vi "Process.vi"(8 "error in":errorcluster, 11 "Sequence Experiment UI":refnum<class "Sequence Experiment UI.lvclass">) -> (0 "error out":errorcluster, 3 "Sequence Experiment UI out":refnum<class "Sequence Experiment UI.lvclass">)   [LabVIEW 2019, in "Sequence Experiment UI.lvclass"]
doc: "---------------------------------------------------------------\nJKI State Machine Objects™\nhttp://jki.net/state-machine-objects/\nCopyright (C) 2005-2015, JKI <info@jki.net>\nALL RIGHTS RESERVEDJKI State Machine Objects (SMO) 1.0.0.5\nJKI - JKI\nCopyright (c) 2016, JKI"
uses:
  Sequence Experiment UI.lvclass
  <vilib>/JKI/JKI SMO/SMO/SMO.lvclass
  <vilib>/JKI/JKI SMO/SMO.UI/SMO.UI.lvclass
  <userlib>/LevyLab/Instrument Framework/SMOs/Instrument/Instrument.lvclass
  C:/Program Files (x86)/National Instruments/LabVIEW 2019/user.lib/LevyLab/Instrument Framework/SMOs/Instrument UI/Instrument UI.lvclass
  C:/Program Files (x86)/National Instruments/LabVIEW 2019/vi.lib/JKI/JKI SMO/SMO.UI/SMO.UI.lvclass
  C:/Program Files (x86)/National Instruments/LabVIEW 2019/vi.lib/JKI/JKI SMO/SMO/SMO.lvclass
  <userlib>/LevyLab/Instrument Framework/SMOs/Instrument UI/Instrument UI.lvclass
  8548cf1d-4249-4658-ae96-b7b094251154.vi
panel:
  out "Numeric":u32
  out "Instrument Response":dbl
  in  "Set Parameter":bool
  in  "Parameter":dbl
  in  "STOP":bool
  out "SMO string":string
  out "SMO Boolean":bool
  out "Logger SMO":dbl
  out "Levy 1":dbl
  # "#todo\nmake UI here. maybe include a nice picture of the hardware?"
  # "#todo\nadd buttons to do stuff (e.g., change a setting)\nButtons should trigger an event"
  # "#todo\nresize this box if you want your UI to be different size"
  # "SMO UI Template"
  # "For instructions on how to use the JKI State Machine Objects, examples and video tutorials, visit:\nhttp://jki.net/state-machine-objects/\n\nJKI State Machine Objects™\nhttp://jki.net/state-machine-objects/\nCopyright (C) 2005-2015, JKI <info@jki.net>\nALL RIGHTS RESERVED"
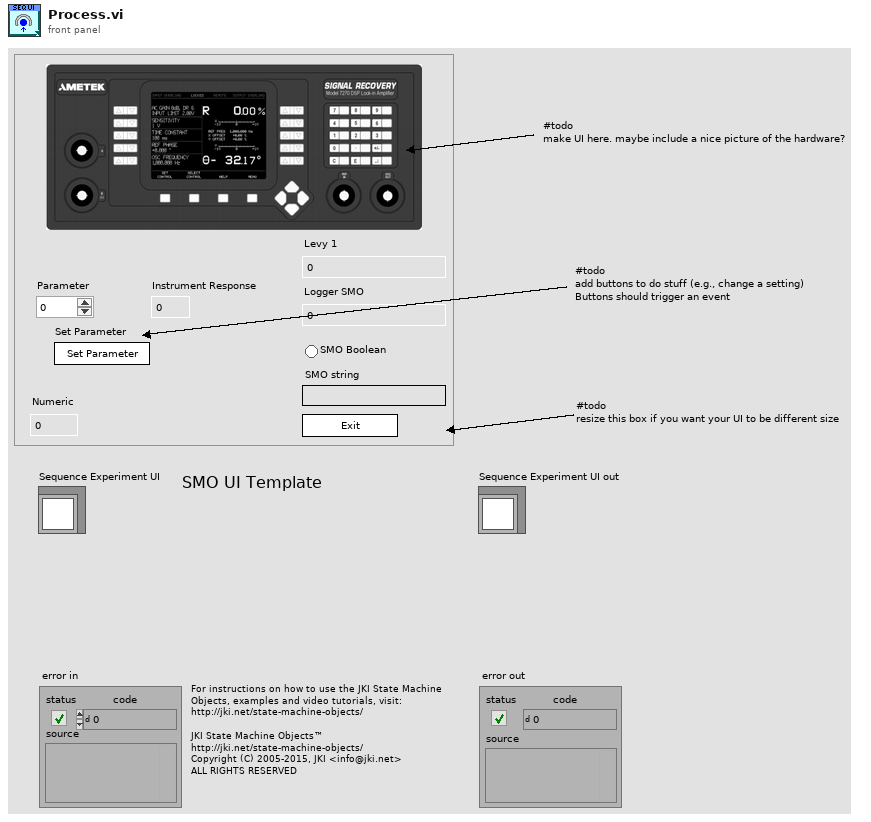
[diagram p1: front panel]
types:
  T1 = enum32{"invalid app kind", "Development System", "Run Time System", "Student Edition", "Embedded LabVIEW", "Evaluation", "Custom"}
  T2 = enum32{"Invalid", "Standard", "Closed", "Hidden", "Minimized", "Maximized"}
  T3 = cluster{"Core":cluster{"Current VI Reference":refnum<vi>, "Close Panel on Exit?":bool, "error":errorcluster}, "Instrument UI":refnum<class "Sequence Experiment UI.lvclass">, "Instrument":refnum<class "Instrument.lvclass">, "getAll":cluster{"Levy 1":dbl, "Logger SMO":dbl, "SMO Boolean":bool, "SMO String":string}, "Parameter":dbl}
  T4 = cluster{"Levy 1":dbl, "Logger SMO":dbl, "SMO Boolean":bool, "SMO String":string}
  T5 = cluster{"Current VI Reference":refnum<vi>, "Close Panel on Exit?":bool, "error":errorcluster}
  T6 = typedef "SMO.lvclass/Protected Events.ctl" = cluster{"StopProcesses":refnum<user-event>, "AbortProcesses":refnum<user-event>, "Config Changed":refnum<user-event>, "Dependency":refnum<user-event>}
  T7 = typedef "Instrument.lvclass/PublicEvents--Cluster.ctl" = cluster{"MessageFromProcess":refnum<user-event>}
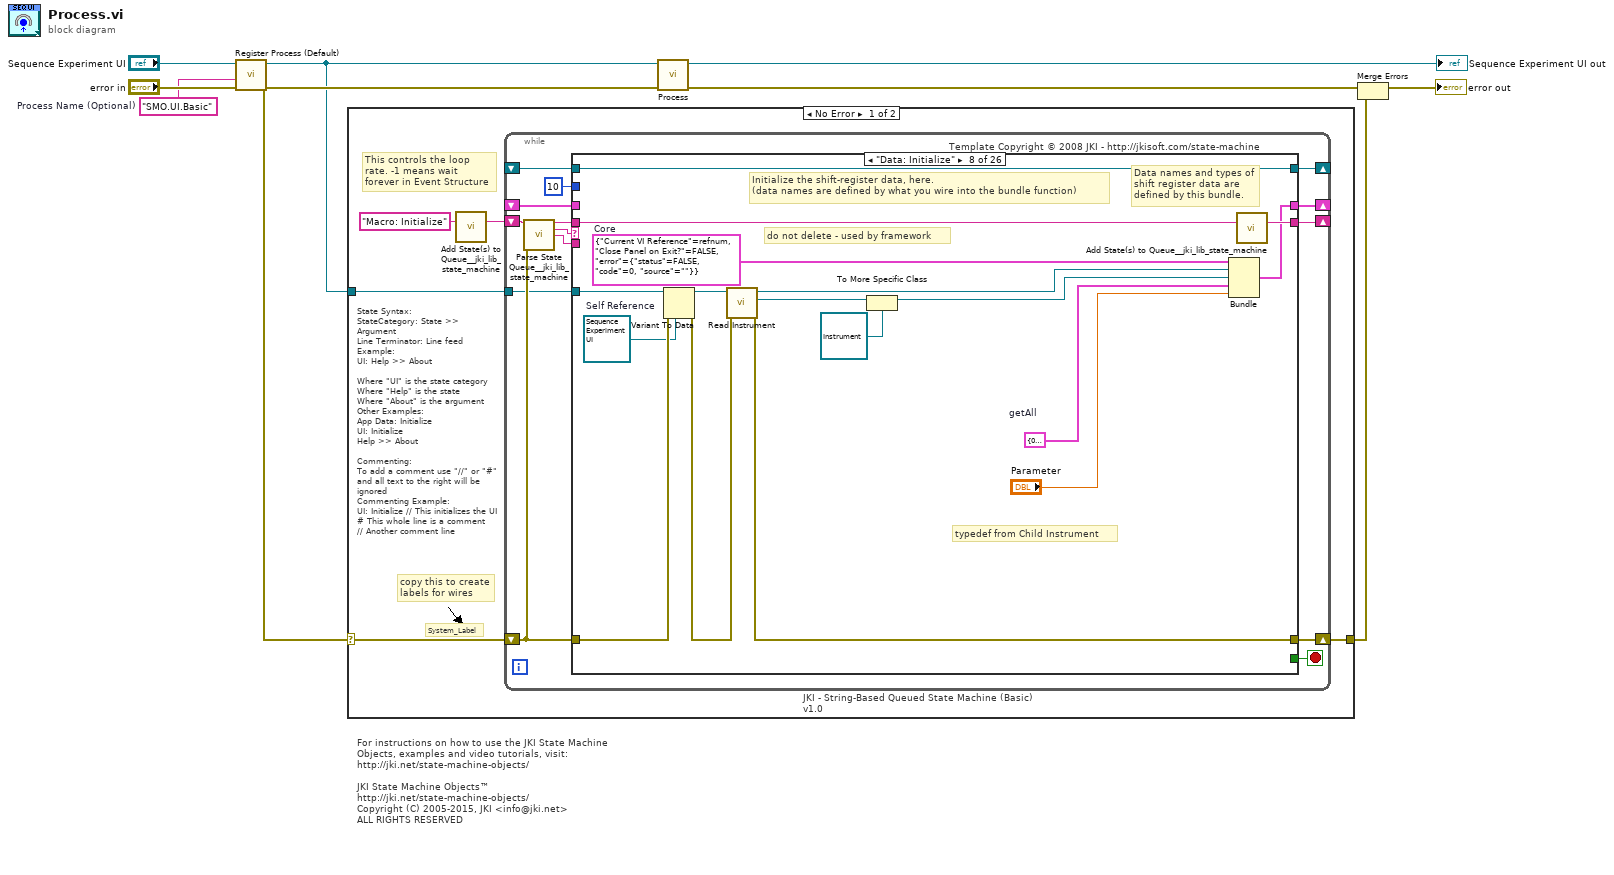
[diagram p0: block diagram]
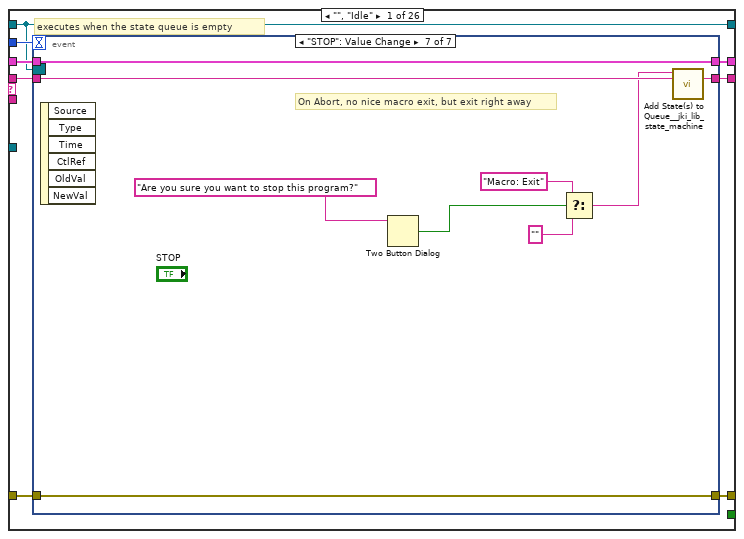
[diagram p2: hidden frame]
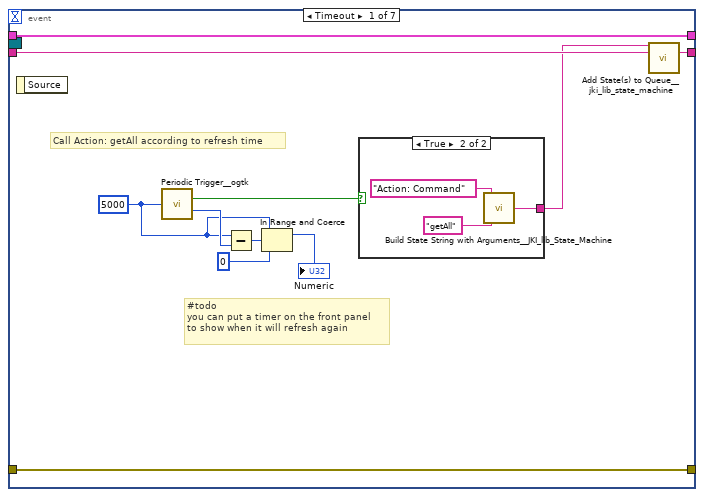
[diagram p3: hidden frame]
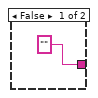
[diagram p4: hidden frame]
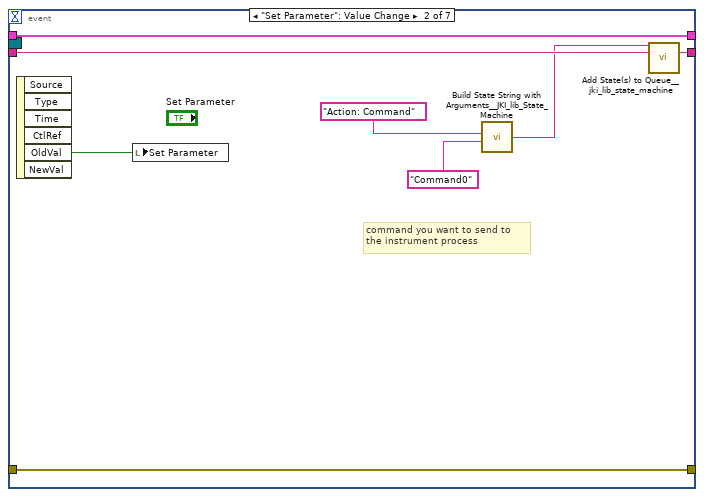
[diagram p5: hidden frame]
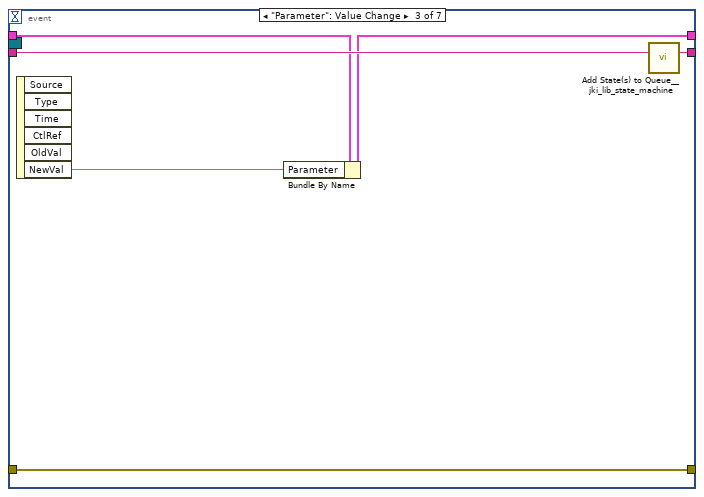
[diagram p6: hidden frame]
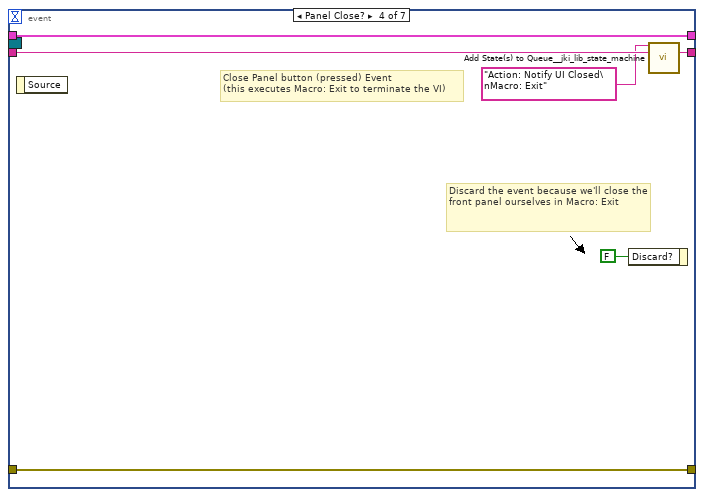
[diagram p7: hidden frame]
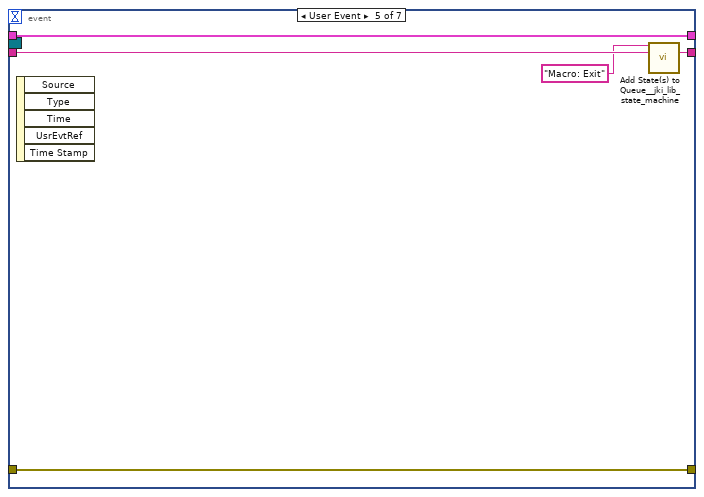
[diagram p8: hidden frame]
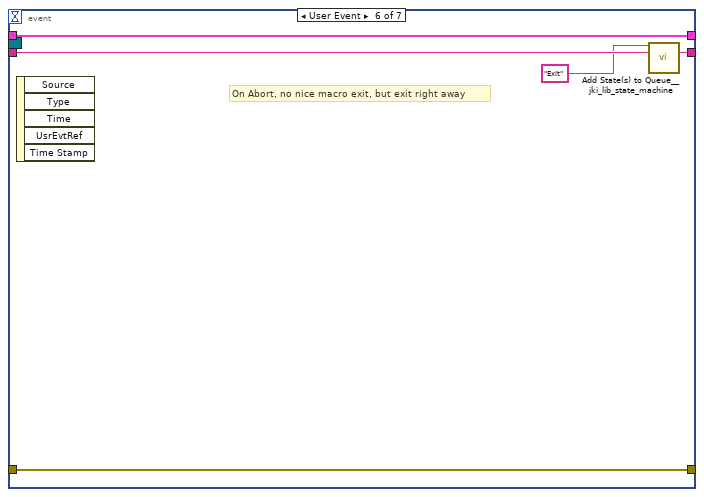
[diagram p9: hidden frame]
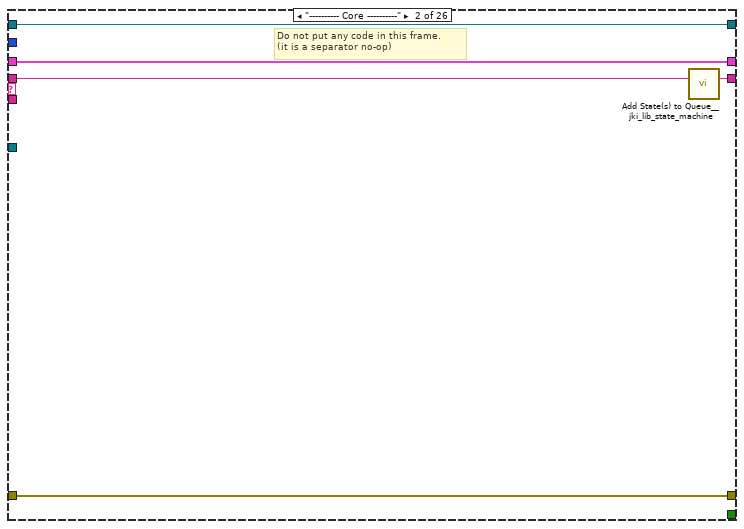
[diagram p10: hidden frame]
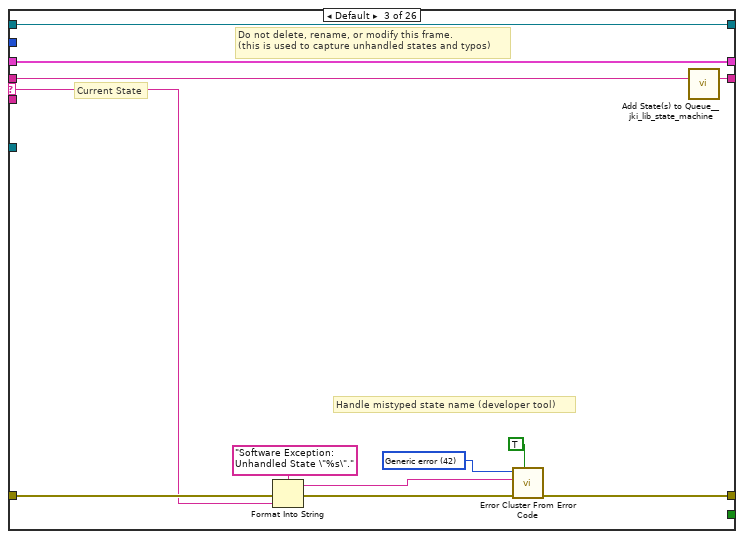
[diagram p11: hidden frame]
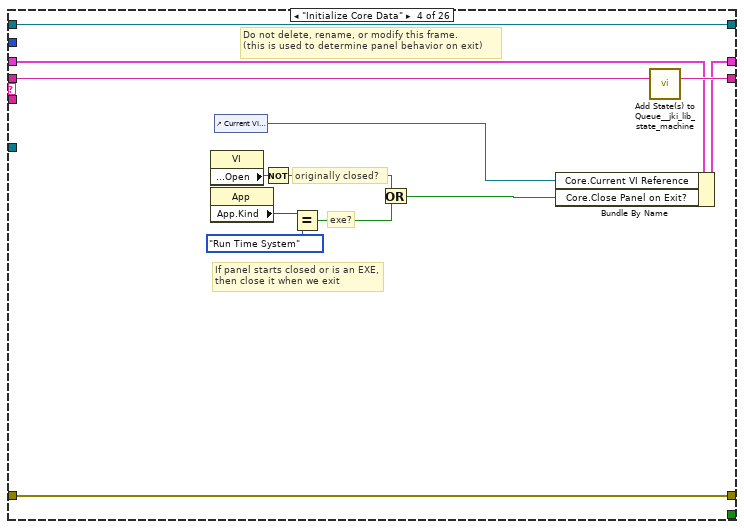
[diagram p12: hidden frame]
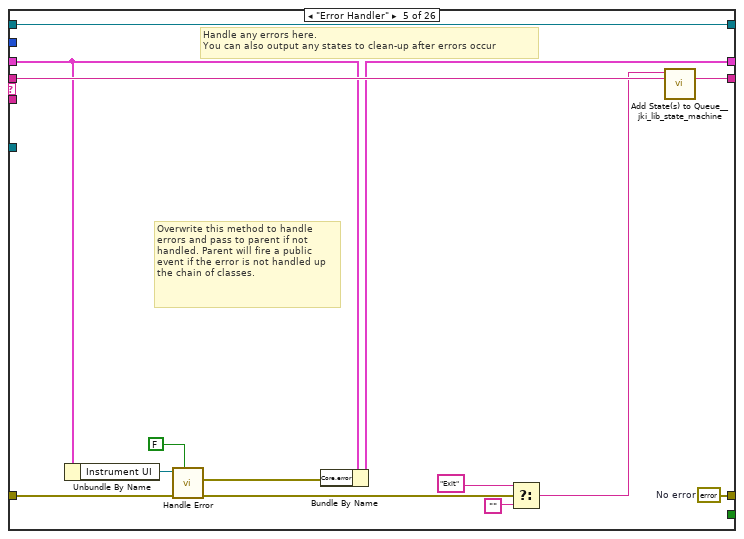
[diagram p13: hidden frame]
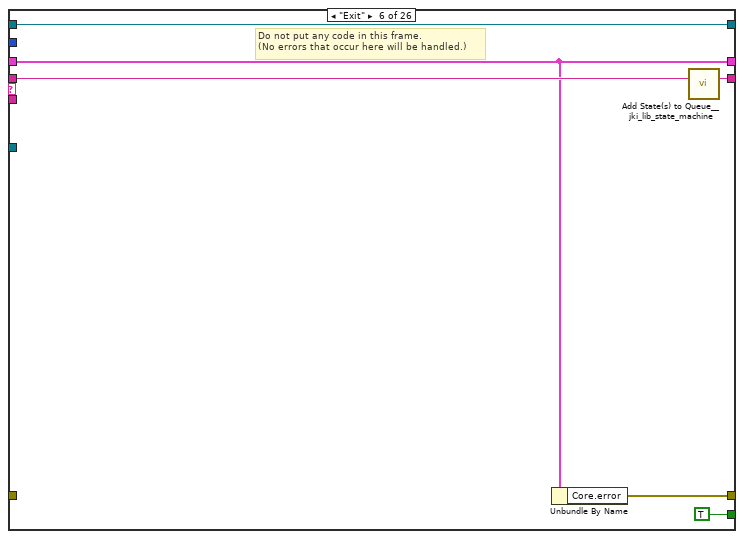
[diagram p14: hidden frame]
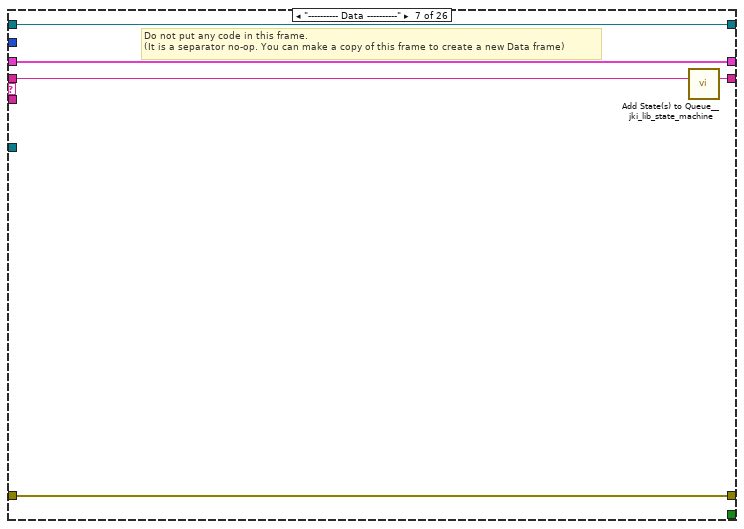
[diagram p15: hidden frame]
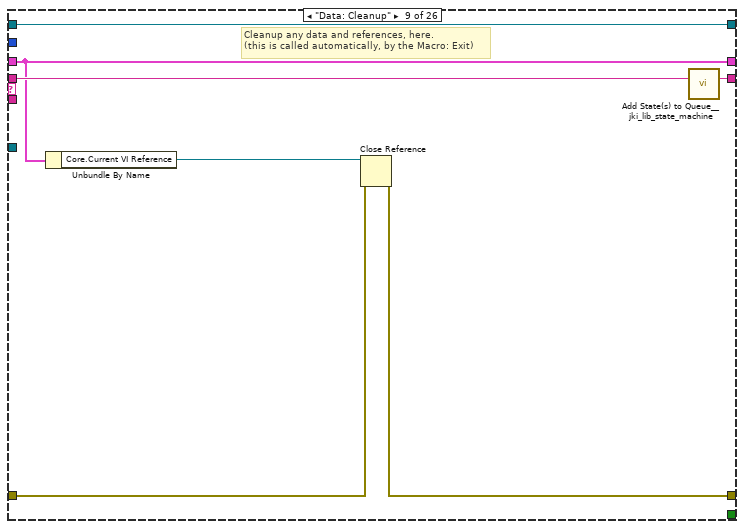
[diagram p16: hidden frame]
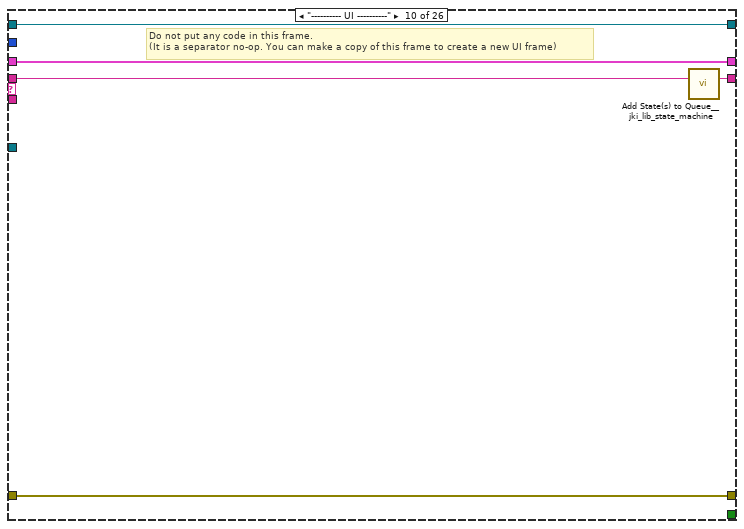
[diagram p17: hidden frame]
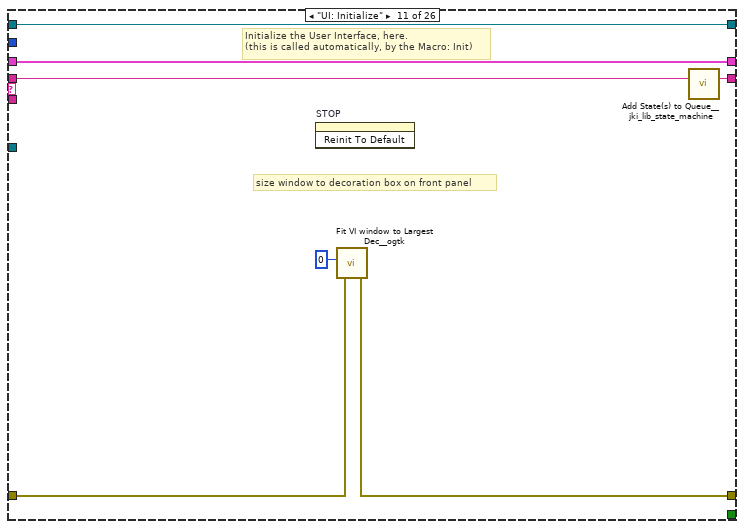
[diagram p18: hidden frame]
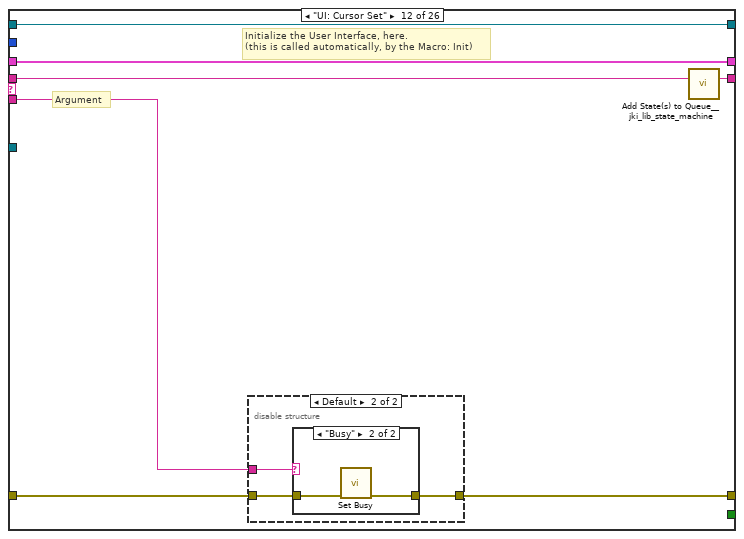
[diagram p19: hidden frame]
diagram:
  w1 = "SMO.UI.Basic"  # Process Name (Optional)
  # "For instructions on how to use the JKI State Machine Objects, examples and video tutorials, visit:\nhttp://jki.net/state-machine-objects/\n\nJKI State Machine Objects™\nhttp://jki.net/state-machine-objects/\nCopyright (C) 2005-2015, JKI <info@jki.net>\nALL RIGHTS RESERVED"
  n1 = call <vilib>:"Register Process (Default).vi"("error in (no error)"="error in", "Process Name (optional)"=w1, "SMO"="Sequence Experiment UI") -> ("error out"=w6:errorcluster, "SelfRef"=w5:refnum<class "Sequence Experiment UI.lvclass">)  [unwired: 7 in]
  n2 = case shown="No Error" w6 {
    selector: w6 -> [w11 w362]
    tunnel: w5 -> [w12 _]
    tunnel: [w10 w362] -> w2
    frame No Error {
      # "State Syntax:\nStateCategory: State >> Argument\nLine Terminator: Line feed\nExample:\nUI: Help >> About\n\nWhere \"UI\" is the state category\nWhere \"Help\" is the state\nWhere \"About\" is the argument\nOther Examples:\nApp Data: Initialize\nUI: Initialize\nHelp >> About\n\nCommenting:\nTo add a comment use \"//\" or \"#\" and all text to the right will be ignored\nCommenting Example:\nUI: Initialize // This initializes the UI\n# This whole line is a comment\n// Another comment line"
      # "copy this to create labels for wires"
      # "This controls the loop rate. -1 means wait forever in Event Structure"
      # "System_Label"
      n3 = call <vilib>:"Add State(s) to Queue__jki_lib_state_machine.vi"("State(s) in (\"\")"="Macro: Initialize") -> ("States Out"=w14:string)  [unwired: 14 in]
      n4 = while "JKI - String-Based Queued State Machine (Basic) v1.0" {
        shift-right: [w21] -> _
        shift-left: _ -> [w20]
        shift-right: [w24] -> w10
        shift-left: w11 -> [w18]
        shift-right: [w23] -> _
        shift-left: w14 -> [w25]
        tunnel: w12 -> [w17]
        shift-right: [w16] -> _
        shift-left: _ -> [w15]
        stop <- w22 stop-if-true
        # "Template Copyright © 2008 JKI - http://jkisoft.com/state-machine"
        n5 = call <vilib>:"Parse State Queue__jki_lib_state_machine.vi"("State Queue"=w25, "Error In (no error)"=w18) -> ("Remaining States"=w27:string, "Current State"=w28:string, "Arguments"=w26:string)  [unwired: 11 in]
        n6 = case shown="\"Data: Initialize\"" w28 {
          selector: w28 -> [_ _ w97 _ _ _ _ _ _ _ _ _ _ _ _ _ _ _ _ _ _ _ _ _ _ _]
          tunnel: w27 -> [w36 w95 w101 w120 w134 w140 w145 w162 w169 w174 w181 w188 w204 w236 w245 w259 w264 w275 w282 w287 w300 w306 w313 w320 w330 w341]
          tunnel: w26 -> [_ _ _ _ _ _ _ _ _ _ _ w182 w198 _ _ _ _ _ _ _ _ _ _ _ _ w335]
          tunnel: w20 -> [w34 w92 w99 w111 w123 w136 w142 _ w164 w171 w179 w186 w200 w233 w241 w246 w261 w272 w277 w284 w298 w304 w309 w316 w327 w332]
          tunnel: [w33 w93 w103 w117 w125 w135 w143 w150 w165 w172 w176 w183 w201 w234 w243 w257 w262 w266 w278 w285 w293 w301 w310 w314 w321 w338] -> w24
          tunnel: w18 -> [w32 w93 w102 w117 w130 _ w143 w159 w166 w172 w177 w184 w202 w234 w243 w257 w262 w267 w279 w285 w295 w302 w310 w315 w321 w333]
          tunnel: [w35 w94 w100 w119 w133 w139 w144 w161 w168 w173 w180 w187 w203 w235 w244 w258 w263 w274 w281 w286 w299 w305 w312 w319 w329 w340] -> w23
          tunnel: [_ _ _ _ _ TRUE _ _ _ _ _ _ _ _ _ _ _ _ _ _ _ _ _ _ _ _] -> w22
          tunnel: [w31 w92 w99 w118 w122 w136 w142 w160 w164 w171 w179 w186 w200 w233 w241 w246 w261 w272 w277 w284 w298 w304 w308 w316 w327 w331] -> w21
          tunnel: 10 ("Timeout") -> [w30 _ _ _ _ _ _ _ _ _ _ _ _ _ _ _ _ _ _ _ _ _ _ _ _ _]
          tunnel: w17 -> [_ _ _ _ _ _ _ w157 _ _ _ _ _ _ _ _ _ _ _ _ _ _ _ _ _ _]
          tunnel: [w29 w91 w96 w108 w132 w137 w141 w156 w163 w170 w178 w185 w197 w232 w242 w251 w260 w273 w280 w283 w297 w303 w311 w318 w328 w339] -> w16
          tunnel: w15 -> [w29 w91 w96 w108 w132 w137 w141 w156 w163 w170 w178 w185 w197 w232 w242 w251 w260 w273 w280 w283 _ w303 w311 w318 w328 w339]
          frame "", "Idle" {
            # "executes when the state queue is empty"
            n7 = event shown="[6] \"STOP\": Value Change" {
              selector: w29 -> [_ _ _ _ _ _ _]
              dyn-events: _ -> [_ _ _ _ _ _ _]
              timeout: w30 -> [_ _ _ _ _ _ _]
              tunnel: w36 -> [w47 w59 w65 w71 w76 w81 w90]
              tunnel: [w46 w58 w64 w70 w75 w80 w89] -> w35
              tunnel: w34 -> [w44 w56 w61 w67 w73 w78 w87]
              tunnel: [w45 w57 w63 w66 w74 w79 w88] -> w33
              tunnel: w32 -> [w45 w57 w63 w66 w74 w79 w88]
              tunnel: [w44 w56 w60 w67 w73 w78 w87] -> w31
              event Timeout {
                w38 = u32 5000 ("time (ms)")
                # "#todo\nyou can put a timer on the front panel\nto show when it will refresh again"
                # "Call Action: getAll according to refresh time"
                n8 = event-data() -> ()  [unwired: 1 in, 1 out]
                n9 = call <userlib>:"Periodic Trigger__ogtk.vi"("time (ms)"=w38) -> ("Triggered"=w42:bool, "timer value"=w41:u32)  [unwired: 12 in, 1 out]
                n10 = Subtract(x=w38, y=w41) -> (x-y=w40:u32)
                n11 = In Range and Coerce(upper limit=w38, x=w40, lower limit=u32 0) -> (coerced(x)=→"Numeric":u32)  [unwired: 1 out]
                n12 = case shown="True" w42 {
                  tunnel: ["" ("State(s) in Front (\"\")") w49] -> w43
                  frame False {
                  }
                  frame True {
                    n13 = call <vilib>:"Build State String with Arguments__JKI_lib_State_Machine.vi"("Arguments (\"\")"="getAll" ("State(s) in Front (\"\")"), "State"="Action: Command" ("State(s) in Front (\"\")")) -> ("State with Arguments"=w49:string)  [unwired: 4 in]
                  }
                }
                n14 = call <vilib>:"Add State(s) to Queue__jki_lib_state_machine.vi"("State(s) in Front (\"\")"=w43, "State(s) in (\"\")"=w47) -> ("States Out"=w46:string)  [unwired: 13 in]
              }
              event "Set Parameter": Value Change {
                # "command you want to send to\nthe instrument process"
                n15 = event-data() -> ("OldVal"=w55:bool)  [unwired: 1 in, 5 out]
                n16 = local write "Set Parameter"(w55) -> ()
                n17 = call <vilib>:"Build State String with Arguments__JKI_lib_State_Machine.vi"("Arguments (\"\")"="Command0" ("State(s) in Front (\"\")"), "State"="Action: Command" ("State(s) in Front (\"\")")) -> ("State with Arguments"=w52:string)  [unwired: 4 in]
                n18 = call <vilib>:"Add State(s) to Queue__jki_lib_state_machine.vi"("State(s) in Front (\"\")"=w52, "State(s) in (\"\")"=w59) -> ("States Out"=w58:string)  [unwired: 13 in]
              }
              event "Parameter": Value Change {
                n19 = event-data() -> ("NewVal"=w62:dbl)  [unwired: 1 in, 5 out]
                n20 = Bundle By Name(cluster=w61, "Parameter"=w62) -> (w60:T3)
                n21 = call <vilib>:"Add State(s) to Queue__jki_lib_state_machine.vi"("State(s) in (\"\")"=w65) -> ("States Out"=w64:string)  [unwired: 14 in]
              }
              event Panel Close? {
                # "Discard the event because we'll close the front panel ourselves in Macro: Exit"
                # "Close Panel button (pressed) Event\n(this executes Macro: Exit to terminate the VI)"
                n22 = event-data() -> ()  [unwired: 1 in, 1 out]
                n23 = event-data("Discard?"=FALSE) -> ()  [unwired: 1 in, 1 out]
                n24 = call <vilib>:"Add State(s) to Queue__jki_lib_state_machine.vi"("State(s) in Front (\"\")"="Action: Notify UI Closed\nMacro: Exit", "State(s) in (\"\")"=w71) -> ("States Out"=w70:string)  [unwired: 13 in]
              }
              event User Event {
                n25 = event-data() -> ()  [unwired: 1 in, 5 out]
                n26 = call <vilib>:"Add State(s) to Queue__jki_lib_state_machine.vi"("State(s) in Front (\"\")"="Macro: Exit", "State(s) in (\"\")"=w76) -> ("States Out"=w75:string)  [unwired: 13 in]
              }
              event User Event {
                # "On Abort, no nice macro exit, but exit right away"
                n27 = event-data() -> ()  [unwired: 1 in, 5 out]
                n28 = call <vilib>:"Add State(s) to Queue__jki_lib_state_machine.vi"("State(s) in Front (\"\")"="Exit", "State(s) in (\"\")"=w81) -> ("States Out"=w80:string)  [unwired: 13 in]
              }
              event "STOP": Value Change {
                # "On Abort, no nice macro exit, but exit right away"
                n29 = event-data() -> ()  [unwired: 1 in, 6 out]
                n30 = Two Button Dialog(message="Are you sure you want to stop this program?") -> (T button?=w86:bool)  [unwired: 2 in]
                n31 = Select(t="Macro: Exit", s=w86, f="") -> (s? t:f=w82:string)
                n32 = call <vilib>:"Add State(s) to Queue__jki_lib_state_machine.vi"("State(s) in Front (\"\")"=w82, "State(s) in (\"\")"=w90) -> ("States Out"=w89:string)  [unwired: 13 in]
              }
            }
          }
          frame "---------- Core ----------" {
            # "Do not put any code in this frame.\n(it is a separator no-op)"
            n33 = call <vilib>:"Add State(s) to Queue__jki_lib_state_machine.vi"("State(s) in (\"\")"=w95) -> ("States Out"=w94:string)  [unwired: 14 in]
          }
          frame Default {
            w106 = 42 items=["No error", "Argument error", "Memory is full", "Out of zone", "End of file", "File already open", "Generic file I/O error", "File not found", "File permission error", "Disk is full", "Duplicate path", "Too many files open", "System feature not enabled", "Resource file not found", "Cannot add resource", "Resource not found", "Image not found", "Image memory error", "Pen does not exist", "Config type invalid", "Config token not found", "Config parse error", "Config memory error", "Bad external code format", "Bad external code offset", "External code not present", "Null window", "Destroy window error", "Null menu", "Print aborted", "Bad print record", "Print driver error", "Windows error during printing", "Memory error during printing", "Print dialog error", "Generic print error", "Invalid device refnum", "Device not found", "Device parameter error", "Device unit error", "Cannot open device", "Device call aborted", "Generic error", "Cancelled by user", "Object ID too low", "Object ID too high", "Object not in heap", "Unknown heap", "Unknown object (invalid DefProc)", "Unknown object (DefProc not in table)", "Message out of range", "Invalid (null) method", "Unknown message", "Manager call not supported", "Bad address", "Network operation in progress", "Network operation timed out", "Connection is busy", "Network attribute not supported", "Network error", "Address in use", "System out of memory", "Connection aborted", "Connection refused", "Not connected", "Already connected", "Connection closed", "Initialization error (interapplication manager)", "Bad occurrence", "Wait on unbound occurrence handler", "Occurrence queue overflow", "Datalog type conflict", "Unused", "Unrecognized type (interapplication manager)", "Memory corrupt", "Failed to make temporary DLL", "Old CIN version", "Drag socket not found", "Failed to load drop-object", "Failed to register OLE object", "Failed to release OLE object", "Format specifier type mismatch", "Unknown format specifier", "Too few format specifiers", "Too many format specifiers", "Scan failed", "Newer CIN version", "Error converting to variant", "Runtime menu error", "Password tampered", "Variant attribute not found", "Incompatible variant data type", "Event data is not available", "Event Store is not present", "Occurrence is not found", "Event Queue is not created", "Event info is not available", "Refnum passed is NULL", "Error retrieving Class GUID", "Error retrieving CoClass GUID", "Error retrieving TypeLib GUID.", "Bad built application magic bytes.", "Specific driver is different from the specific driver associated with the Logical Name.", "There is no session opened to the class driver.", "Max Error", "MAX - Error with config objects", "MAX - Error loading configuration", "MAX - Group not supported"]
            # "Current State"
            # "Do not delete, rename, or modify this frame.\n(this is used to capture unhandled states and typos)"
            # "Handle mistyped state name (developer tool)"
            n34 = Format Into String(format string="Software Exception: Unhandled State \"%s\"." ("message"), error in=w102, w97) -> (resulting string=w105:string, error out=w104:errorcluster)  [unwired: 1 in]
            n35 = call <vilib>:"Error Cluster From Error Code.vi"("show call chain? (False)"=TRUE, "error in (no error)"=w104, "error message (\"\")"=w105, "error code (0)"=w106) -> ("error out"=w103:errorcluster)  [unwired: 5 in]
            n36 = call <vilib>:"Add State(s) to Queue__jki_lib_state_machine.vi"("State(s) in (\"\")"=w101) -> ("States Out"=w100:string)  [unwired: 14 in]
          }
          frame "Initialize Core Data" {
            # "Do not delete, rename, or modify this frame.\n(this is used to determine panel behavior on exit)"
            # "originally closed?"
            # "exe?"
            # "If panel starts closed or is an EXE, then close it when we exit"
            n37 = property class="VI"() -> ("Front Panel.Open"=w116:bool)  [unwired: 2 in, 2 out]
            n38 = property class="App"() -> ("App.Kind"=w115:T1)  [unwired: 2 in, 2 out]
            n39 = control-ref of="Current VI Reference"() -> (w109:refnum<vi>)
            n40 = Not(x=w116) -> (.not. x?=w113:bool)
            n41 = Equal?(x=w115, y=T1."Run Time System" ("Application:Kind")) -> (x = y?=w112:bool)
            n42 = Or(x=w113, y=w112) -> (x .or. y?=w110:bool)
            n43 = Bundle By Name(cluster=w111, "Core.Current VI Reference"=w109, "Core.Close Panel on Exit?"=w110) -> (w118:T3)
            n44 = call <vilib>:"Add State(s) to Queue__jki_lib_state_machine.vi"("State(s) in (\"\")"=w120) -> ("States Out"=w119:string)  [unwired: 14 in]
          }
          frame "Error Handler" {
            w125 = errorcluster {"status"=FALSE, "code"=0, "source"=""}  # No error
            # "Overwrite this method to handle errors and pass to parent if not handled. Parent will fire a public event if the error is not handled up the chain of classes."
            # "Handle any errors here.\nYou can also output any states to clean-up after errors occur"
            n45 = Unbundle By Name(w123) -> ("Instrument UI"=w131:refnum<class "Sequence Experiment UI.lvclass">)
            n46 = call-dynamic "Handle Error.vi"("Stop on Unhandled Error (T)"=FALSE, "error in"=w130, "SMO"=w131) -> ("handling error"=w126:errorcluster, "Unhandled error"=w124:errorcluster)  [unwired: 6 in, 1 out]
            n47 = Bundle By Name(cluster=w123, "Core.error"=w124) -> (w122:T3)
            n48 = Select(t="Exit", s=w126, f="") -> (s? t:f=w127:string)
            n49 = call <vilib>:"Add State(s) to Queue__jki_lib_state_machine.vi"("State(s) in Front (\"\")"=w127, "State(s) in (\"\")"=w134) -> ("States Out"=w133:string)  [unwired: 13 in]
          }
          frame "Exit" {
            # "Do not put any code in this frame.\n(No errors that occur here will be handled.)"
            n50 = Unbundle By Name(w136) -> ("Core.error"=w135:errorcluster)
            n51 = call <vilib>:"Add State(s) to Queue__jki_lib_state_machine.vi"("State(s) in (\"\")"=w140) -> ("States Out"=w139:string)  [unwired: 14 in]
          }
          frame "---------- Data ----------" {
            # "Do not put any code in this frame.\n(It is a separator no-op. You can make a copy of this frame to create a new Data frame)"
            n52 = call <vilib>:"Add State(s) to Queue__jki_lib_state_machine.vi"("State(s) in (\"\")"=w145) -> ("States Out"=w144:string)  [unwired: 14 in]
          }
          frame "Data: Initialize" {
            w153 = T4 {"Levy 1"=0.0, "Logger SMO"=0.0, "SMO Boolean"=FALSE, "SMO String"=""}  # getAll
            w155 = T5 {"Current VI Reference"=refnum, "Close Panel on Exit?"=FALSE, "error"={"status"=FALSE, "code"=0, "source"=""}}  # Core
            w158 = refnum<class "Sequence Experiment UI.lvclass"> refnum  # Self Reference
            # "typedef from Child Instrument"
            # "do not delete - used by framework"
            # "Data names and types of shift register data are defined by this bundle."
            # "Initialize the shift-register data, here.\n(data names are defined by what you wire into the bundle function)"
            n53 = Variant To Data(error in=w159, type=w158, Variant=w157) -> (data=w148:refnum<class "Sequence Experiment UI.lvclass">, error out=w151:errorcluster)
            n54 = call <userlib>:"Read Instrument.vi"("error in (no error)"=w151, "Instrument UI in"=w148) -> ("error out"=w150:errorcluster, "Instrument"=w149:refnum<class "Instrument.lvclass">, "Instrument UI"=w147:refnum<class "Sequence Experiment UI.lvclass">)  [unwired: 7 in]
            n55 = To More Specific Class(target class=refnum<class "Instrument.lvclass"> refnum ("Instrument"), reference=w149) -> (specific class reference=w152:refnum<class "Instrument.lvclass">)  [unwired: 1 in, 1 out]
            n56 = Bundle("Core"=w155, "Instrument UI"=w147, "Instrument"=w152, "getAll"=w153, "Parameter"="Parameter") -> (w160:T3)  [unwired: 1 in]
            n57 = call <vilib>:"Add State(s) to Queue__jki_lib_state_machine.vi"("State(s) in (\"\")"=w162) -> ("States Out"=w161:string)  [unwired: 14 in]
          }
          frame "Data: Cleanup" {
            # "Cleanup any data and references, here.\n(this is called automatically, by the Macro: Exit)"
            n58 = Unbundle By Name(w164) -> ("Core.Current VI Reference"=w167:refnum<vi>)
            n59 = Close Reference(reference=w167, error in (no error)=w166) -> (error out=w165:errorcluster)
            n60 = call <vilib>:"Add State(s) to Queue__jki_lib_state_machine.vi"("State(s) in (\"\")"=w169) -> ("States Out"=w168:string)  [unwired: 14 in]
          }
          frame "---------- UI ----------" {
            # "Do not put any code in this frame.\n(It is a separator no-op. You can make a copy of this frame to create a new UI frame)"
            n61 = call <vilib>:"Add State(s) to Queue__jki_lib_state_machine.vi"("State(s) in (\"\")"=w174) -> ("States Out"=w173:string)  [unwired: 14 in]
          }
          frame "UI: Initialize" {
            # "size window to decoration box on front panel"
            # "Initialize the User Interface, here.\n(this is called automatically, by the Macro: Init)"
            n62 = invoke on="STOP" class="Bool (strict)" method="Reinit To Default"() -> ()  [unwired: 3 in, 3 out]
            n63 = call <userlib>:"Fit VI window to Largest Dec__ogtk.vi"("error in (no error)"=w177, "border spacing (2 px)"=0) -> ("error out"=w176:errorcluster)  [unwired: 4 in, 1 out]
            n64 = call <vilib>:"Add State(s) to Queue__jki_lib_state_machine.vi"("State(s) in (\"\")"=w181) -> ("States Out"=w180:string)  [unwired: 14 in]
          }
          frame "UI: Cursor Set" {
            # "Argument"
            # "Initialize the User Interface, here.\n(this is called automatically, by the Macro: Init)"
            n65 = disable-structure shown="Default" {
              disable-tunnel: w184 -> [w189 w192]
              disable-tunnel: [w189 w191] -> w183
              disable-tunnel: w182 -> [_ w190]
              frame condition #0 {
              }
              frame condition #1 (active) {
                n66 = case shown="\"Busy\"" w190 {
                  tunnel: w192 -> [w194 w196]
                  tunnel: [w193 w195] -> w191
                  frame "Idle", Default {
                    n67 = call <vilib>:"Unset Busy.vi"("error in (no error)"=w194) -> ("error out"=w193:errorcluster)  [unwired: 10 in]
                  }
                  frame "Busy" {
                    n68 = call <vilib>:"Set Busy.vi"("error in (no error)"=w196) -> ("error out"=w195:errorcluster)  [unwired: 9 in, 1 out]
                  }
                }
              }
            }
            n69 = call <vilib>:"Add State(s) to Queue__jki_lib_state_machine.vi"("State(s) in (\"\")"=w188) -> ("States Out"=w187:string)  [unwired: 14 in]
          }
          frame "UI: Front Panel State" {
            # "Argument"
            # "Set Front Panel Open or Closed\n(Usage: \"UI: Front Panel State >> Open|Close\")"
            n70 = Unbundle By Name(w200) -> ("Core.Current VI Reference"=w199:refnum<vi>)
            n71 = disable-structure shown="Default" {
              disable-tunnel: w202 -> [w208 w231]
              disable-tunnel: [w207 w231] -> w201
              disable-tunnel: w199 -> [w206 _]
              disable-tunnel: w198 -> [w205 _]
              frame condition #0 (active) {
                n72 = case shown="\"Close\"" w205 {
                  tunnel: w208 -> [w212 w225]
                  tunnel: [w214 w226] -> w207
                  tunnel: w206 -> [w213 w223]
                  frame "Open", Default {
                    n73 = property class="VI"(reference=w213, error in=w212) -> (reference out=w210:refnum<vi>, error out=w211:errorcluster, "FP.State"=w209:T2)
                    n74 = case shown="\"Closed\"" w209 {
                      tunnel: [w217 w220] -> w214
                      tunnel: w211 -> [w216 w220]
                      tunnel: w210 -> [w215 _]
                      frame "Closed" {
                        n75 = invoke class="VI" method="FP.Open"(reference=w215, error in=w216, "Activate"=TRUE, "State"=T2."Standard") -> (error out=w217:errorcluster)  [unwired: 1 in, 4 out]
                      }
                      frame Default {
                      }
                    }
                  }
                  frame "Close" {
                    n76 = property class="VI"(reference=w223, error in=w225) -> (reference out=w222:refnum<vi>, error out=w224:errorcluster, "FP.State"=w221:T2)
                    n77 = case shown="Default" w221 {
                      tunnel: [w227 w230] -> w226
                      tunnel: w224 -> [w227 w229]
                      tunnel: w222 -> [_ w228]
                      frame "Invalid", "Closed" {
                      }
                      frame Default {
                        n78 = invoke class="VI" method="FP.Close"(reference=w228, error in=w229) -> (error out=w230:errorcluster)  [unwired: 1 in, 2 out]
                      }
                    }
                  }
                }
              }
              frame condition #1 {
              }
            }
            n79 = call <vilib>:"Add State(s) to Queue__jki_lib_state_machine.vi"("State(s) in (\"\")"=w204) -> ("States Out"=w203:string)  [unwired: 14 in]
          }
          frame "---------- Macro ----------" {
            # "Do not put any code in this frame.\n(It is a separator no-op. You can make a copy of this frame to create a new Macro frame)"
            n80 = call <vilib>:"Add State(s) to Queue__jki_lib_state_machine.vi"("State(s) in (\"\")"=w236) -> ("States Out"=w235:string)  [unwired: 14 in]
          }
          frame "Macro: Initialize" {
            w239 = "UI: Initialize\n//UI: Front Panel State >> Open"  # UI: Initialize //UI: Front Panel State >> Open
            # "Initialization Macro\n(This is called once, when the VI starts)"
            n81 = call <vilib>:"Add State(s) to Queue__jki_lib_state_machine.vi"("State(s) in Front (\"\")"="Data: Initialize\nInitialize Core Data\nEvents: Register", "State(s) in (\"\")"="Process: Sync", "State(s) at Back (\"\")"=w239) -> ("States Out"=w238:string)  [unwired: 12 in]
            n82 = call <vilib>:"Add State(s) to Queue__jki_lib_state_machine.vi"("State(s) in Front (\"\")"=w238, "State(s) in (\"\")"=w245) -> ("States Out"=w244:string)  [unwired: 13 in]
          }
          frame "Macro: Exit" {
            # "Exit Macro\n(This is called once, when the VI exits)"
            n83 = Unbundle By Name(w246) -> ("Core.Close Panel on Exit?"=w256:bool)
            n84 = Select(t="UI: Front Panel State >> Close", s=w256, f="") -> (s? t:f=w253:string)
            n85 = call <vilib>:"Add State(s) to Queue__jki_lib_state_machine.vi"("State(s) in Front (\"\")"="Data: Cleanup\nEvents: Unregister\nProcess: Self Terminate", "State(s) in (\"\")"="Process: Sync", "State(s) at Back (\"\")"="Exit") -> ("States Out"=w248:string)  [unwired: 12 in]
            n86 = call <vilib>:"Add State(s) to Queue__jki_lib_state_machine.vi"("State(s) in (\"\")"=w253, "State(s) at Back (\"\")"=w248) -> ("States Out"=w252:string)  [unwired: 13 in]
            n87 = call <vilib>:"Add State(s) to Queue__jki_lib_state_machine.vi"("State(s) in Front (\"\")"=w252, "State(s) in (\"\")"=w259) -> ("States Out"=w258:string)  [unwired: 13 in]
          }
          frame "---------- Process ----------" {
            # "Template Separator\n(You can make a copy of, or modify, this frame)"
            n88 = call <vilib>:"Add State(s) to Queue__jki_lib_state_machine.vi"("State(s) in (\"\")"=w264) -> ("States Out"=w263:string)  [unwired: 14 in]
          }
          frame "Process: Sync" {
            n89 = Unbundle By Name(w272) -> ("Instrument UI"=w268:refnum<class "Sequence Experiment UI.lvclass">)
            n90 = call <vilib>:"WaitOnProcessSync.vi"("error in (no error)"=w267, "SMO"=w268) -> ("error out"=w266:errorcluster, "Don't run?"=w271:bool)  [unwired: 7 in, 1 out]
            n91 = Select(t="Data: Cleanup\nEvents: Unregister\nExit", s=w271, f="") -> (s? t:f=w265:string)
            n92 = call <vilib>:"Add State(s) to Queue__jki_lib_state_machine.vi"("State(s) in Front (\"\")"=w265, "State(s) in (\"\")"=w275) -> ("States Out"=w274:string)  [unwired: 13 in]
          }
          frame "Process: Self Terminate" {
            n93 = Unbundle By Name(w277) -> ("Instrument UI"=w276:refnum<class "Sequence Experiment UI.lvclass">)
            n94 = call <vilib>:"SelfTerminate.vi"("error in (no error)"=w279, "SMO in"=w276) -> ("error out"=w278:errorcluster)  [unwired: 8 in, 1 out]
            n95 = call <vilib>:"Add State(s) to Queue__jki_lib_state_machine.vi"("State(s) in (\"\")"=w282) -> ("States Out"=w281:string)  [unwired: 14 in]
          }
          frame "---------- Events ----------" {
            # "Template Separator\n(You can make a copy of, or modify, this frame)"
            n96 = call <vilib>:"Add State(s) to Queue__jki_lib_state_machine.vi"("State(s) in (\"\")"=w287) -> ("States Out"=w286:string)  [unwired: 14 in]
          }
          frame "Events: Register" {
            # "Expand to add\nmore events"
            # "Base Class Protected Events"
            n97 = Unbundle By Name(w298) -> ("Instrument UI"=w288:refnum<class "Sequence Experiment UI.lvclass">, "Instrument"=w291:refnum<class "Instrument.lvclass">)
            n98 = call <vilib>:"GetProtectedEvents.vi"("SMO"=w288) -> ("error out"=w292:errorcluster, "SMO Protected Events"=w296:T6)  [unwired: 8 in, 1 out]
            n99 = call <userlib>:"Instrument.GetPublicEvents.vi"("Instrument"=w291) -> ("error out"=w289:errorcluster, "Instrument Public Events"=w290:T7)  [unwired: 8 in, 1 out]
            n100 = register-events(w296, w290) -> (reference out=w297:refnum<event-registration>, error out=w294:errorcluster)  [unwired: 2 in]
            n101 = Merge Errors(w289, w295, w294, w292) -> (w293:errorcluster)
            n102 = call <vilib>:"Add State(s) to Queue__jki_lib_state_machine.vi"("State(s) in (\"\")"=w300) -> ("States Out"=w299:string)  [unwired: 14 in]
          }
          frame "Events: Unregister" {
            n103 = Unregister For Events(event registration refnum=w303, error in=w302) -> (error out=w301:errorcluster)
            n104 = call <vilib>:"Add State(s) to Queue__jki_lib_state_machine.vi"("State(s) in (\"\")"=w306) -> ("States Out"=w305:string)  [unwired: 14 in]
          }
          frame "---------- Action ----------" {
            n105 = Unbundle By Name(w309) -> ("Instrument UI"=w307:refnum<class "Sequence Experiment UI.lvclass">)
            n106 = Bundle By Name(cluster=w309, "Instrument UI"=w307) -> (w308:T3)
            n107 = call <vilib>:"Add State(s) to Queue__jki_lib_state_machine.vi"("State(s) in (\"\")"=w313) -> ("States Out"=w312:string)  [unwired: 14 in]
          }
          frame "Action: Notify UI Closed" {
            # "Notify that the UI has been closed"
            n108 = Unbundle By Name(w316) -> ("Instrument UI"=w317:refnum<class "Sequence Experiment UI.lvclass">)
            n109 = call <vilib>:"Hide.vi"("error in (no error)"=w315, "SMO.UI"=w317) -> ("error out"=w314:errorcluster)  [unwired: 8 in, 1 out]
            n110 = call <vilib>:"Add State(s) to Queue__jki_lib_state_machine.vi"("State(s) in (\"\")"=w320) -> ("States Out"=w319:string)  [unwired: 14 in]
          }
          frame "Action: Update Front Panel" {
            # "do this way to have nicer UI or only display what you want"
            n111 = Unbundle By Name(w327) -> ("getAll"=w322:T4)
            n112 = Unbundle By Name(w322) -> ("Levy 1"=→"Levy 1":dbl, "Logger SMO"=→"Logger SMO":dbl, "SMO Boolean"=→"SMO Boolean":bool, "SMO String"=→"SMO string":string)
            n113 = call <vilib>:"Add State(s) to Queue__jki_lib_state_machine.vi"("State(s) in (\"\")"=w330) -> ("States Out"=w329:string)  [unwired: 14 in]
          }
          frame "Action: Command" {
            # "command"
            n114 = Unbundle By Name(w332) -> ("Instrument"=w336:refnum<class "Instrument.lvclass">, "Parameter"=w334:dbl)
            n115 = case shown="\"getAll\"" w335 {
              tunnel: w334 -> [_ _ w361]
              tunnel: w333 -> [w344 w351 w359]
              tunnel: [w344 w349 w355] -> w338
              tunnel: ["" ("State(s) in Front (\"\")") "Action: Update Front Panel" ("State(s) in Front (\"\")") "" ("State(s) in Front (\"\")")] -> w337
              tunnel: w336 -> [_ w352 _]
              tunnel: w332 -> [w342 w348 w356]
              tunnel: [w342 w353 w356] -> w331
              frame Default {
              }
              frame "getAll" {
                n116 = Unbundle By Name(w348) -> ("getAll"=w347:T4)
                n117 = call "GET ALL.vim"("error in (no error)"=w351, "Instrument in"=w352) -> ("error out"=w350:errorcluster, "getAll"=w345:variant)  [unwired: 7 in, 1 out]
                n118 = Variant To Data(error in=w350, type=w347, Variant=w345) -> (data=w346:T4, error out=w349:errorcluster)
                n119 = Bundle By Name(cluster=w348, "getAll"=w346) -> (w353:T3)
              }
              frame "Command0" {
                n120 = Variant To Data(error in=w359, type=0.0 ("Magnet Return"), Variant=w361) -> (data=→"Instrument Response":dbl, error out=w355:errorcluster)
              }
            }
            n121 = call <vilib>:"Add State(s) to Queue__jki_lib_state_machine.vi"("State(s) in Front (\"\")"=w337, "State(s) in (\"\")"=w341) -> ("States Out"=w340:string)  [unwired: 13 in]
          }
        }
      }
    }
    frame Error {
    }
  }
  n122 = call-parent "Process.vi"("error in"=w6, "Instrument UI in"=w5) -> ("error out"=w3:errorcluster, "Instrument UI out"=→"Sequence Experiment UI out":refnum<class "Sequence Experiment UI.lvclass">)  [unwired: 8 in]
  n123 = Merge Errors(w3, w2) -> (→"error out":errorcluster)
